vi "RichToFlatcif_manager_PluginType.vi"(5 "OutputClusterType":T1, 11 "InputCluster":T4) -> (3 "OutputCluster":T1)   [LabVIEW 2021, in "CIF_Manager_client.lvlib"]
uses:
  cif_manager_PluginType.ctl
  cif_common_ShortVersion.ctl
  cif_management_common_PluginMetadata.ctl
  cif_manager_PluginType_Flat.ctl
  cif_common_ShortVersion_Flat.ctl
  cif_management_common_PluginMetadata_Flat.ctl
  CIF_Manager_client.lvlib
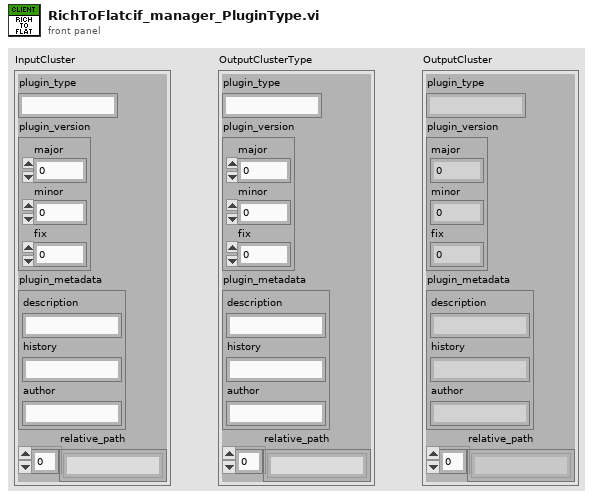
[diagram p1: front panel]
types:
  T1 = typedef "CIF_Manager_client.lvlib/cif_manager_PluginType_Flat.ctl" = cluster{"plugin_type":string, "plugin_version":T2, "plugin_metadata":T3, "relative_path":string[]}
  T2 = typedef "CIF_Manager_client.lvlib/cif_common_ShortVersion_Flat.ctl" = cluster{"major":u32, "minor":u32, "fix":u32}
  T3 = typedef "CIF_Manager_client.lvlib/cif_management_common_PluginMetadata_Flat.ctl" = cluster{"description":string, "history":string, "author":string}
  T4 = typedef "CIF_Manager_client.lvlib/cif_manager_PluginType.ctl" = cluster{"plugin_type":string, "plugin_version":T5, "plugin_metadata":T6, "relative_path":string[]}
  T5 = typedef "CIF_Manager_client.lvlib/cif_common_ShortVersion.ctl" = cluster{"major":u32, "minor":u32, "fix":u32}
  T6 = typedef "CIF_Manager_client.lvlib/cif_management_common_PluginMetadata.ctl" = cluster{"description":string, "history":string, "author":string}
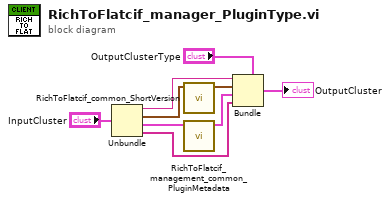
[diagram p0: block diagram]
diagram:
  n1 = Unbundle "Unbundle"("InputCluster") -> ("plugin_type"=w6:string, "plugin_version"=w5:T5, "plugin_metadata"=w3:T6, "relative_path"=w1:string[])
  n2 = call "RichToFlatcif_common_ShortVersion.vi"("InputCluster"=w5) -> ("OutputCluster"=w4:T2)  [unwired: 10 in]
  n3 = call "RichToFlatcif_management_common_PluginMetadata.vi"("InputCluster"=w3) -> ("OutputCluster"=w2:T3)  [unwired: 10 in]
  n4 = Bundle "Bundle"(cluster="OutputClusterType", "plugin_type"=w6, "plugin_version"=w4, "plugin_metadata"=w2, "relative_path"=w1) -> (→"OutputCluster":T1)
